vi "Globals.vi"() -> ()   [LabVIEW 2020, in "OperateExcel.lvlib"]
uses:
  OperateExcel.lvlib
panel:
  out "引用簇":T1
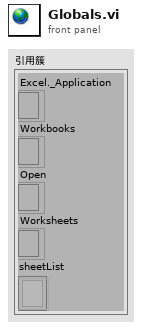
[diagram p1: front panel]
types:
  T1 = typedef "OperateExcel.lvlib/引用簇.ctl" = cluster{"Excel._Application":refnum<k7>, "Workbooks":refnum<k7>, "Open":refnum<k7>, "Worksheets":refnum<k7>, "sheetList":refnum<k7>[]}
diagram:
